vi "ctx autoconfigure devices and accesspoint5.vi"(0 "context":u32, 1 "accel_full_scale_mode":bool, 2 "enable_gyro":bool, 3 "decimation_rate":u32(ring) items=["APDM_DECIMATE_1x1", "APDM_DECIMATE_2x1", "APDM_DECIMATE_2x2", "APDM_DECIMATE_5x1", "APDM_DECIMATE_4x2", "APDM_DECIMATE_5x2", "APDM_DECIMATE_4x4", "APDM_DECIMATE_5x4", "APDM_DECIMATE_8x4", "APDM_DECIMATE_8x5", "APDM_DECIMATE_8x8"], 5 "wireless_channel_number":u8, 7 "enable_sd_card":bool, 9 "erase_sd_card":bool, 12 "enable_accel":bool, 13 "enable_mag":bool) -> (4 "context out":u32, 6 "function return":i32)   [LabVIEW 2019, in "apdm.lvlib"]
doc: "APDM_EXPORT int apdm_ctx_autoconfigure_devices_and_accesspoint5(apdm_ctx_t context, const uint8_t wireless_channel_number, const bool enable_sd_card,\n const bool erase_sd_card, const bool accel_full_scale_mode, const bool enable_accel, const bool enable_gyro, const bool enable_mag, const apdm_monitor_decimation_rate_t decimation_rate);"
uses:
  apdm.lvlib
  Lee Lab/CP FES Walking 2018/Code/Working/LabVIEW/apdm.dll
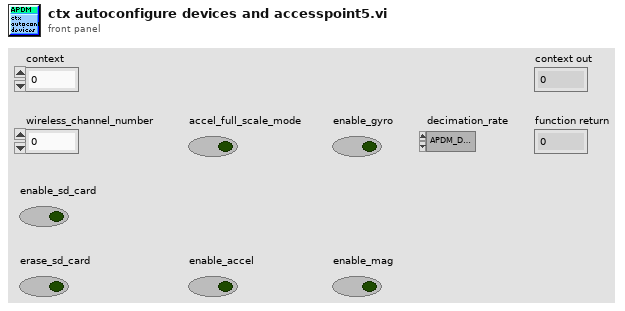
[diagram p1: front panel]
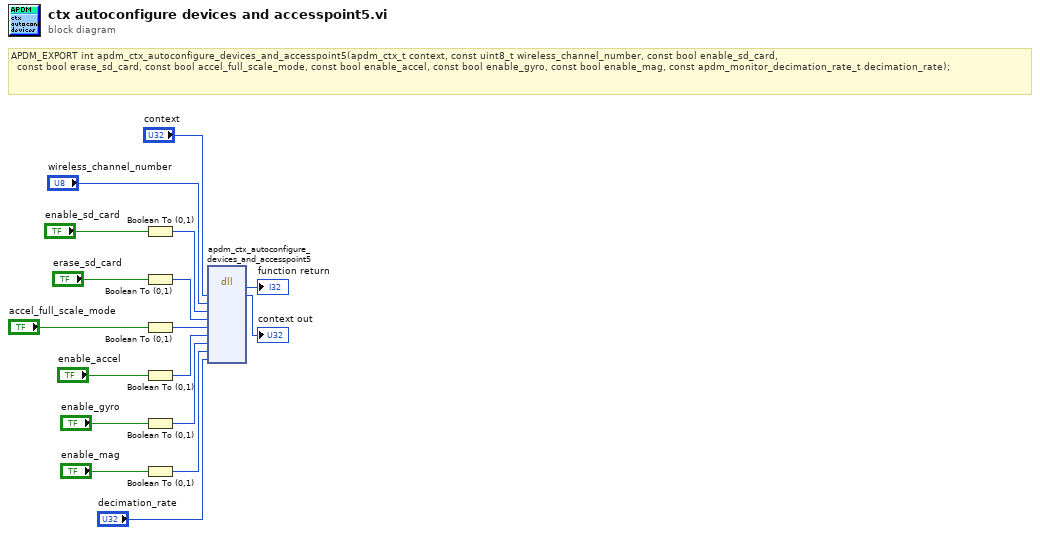
[diagram p0: block diagram]
diagram:
  # "APDM_EXPORT int apdm_ctx_autoconfigure_devices_and_accesspoint5(apdm_ctx_t context, const uint8_t wireless_channel_number, const bool enable_sd_card,\n\t\tconst bool erase_sd_card, const bool accel_full_scale_mode, const bool enable_accel, const bool enable_gyro, const bool enable_mag, const apdm_monitor_decimation_rate_t decimation_rate);"
  n1 = Boolean To (0,1)(Boolean="enable_sd_card") -> (0, 1=w12:i16)
  n2 = Boolean To (0,1)(Boolean="erase_sd_card") -> (0, 1=w10:i16)
  n3 = Boolean To (0,1)(Boolean="accel_full_scale_mode") -> (0, 1=w8:i16)
  n4 = Boolean To (0,1)(Boolean="enable_accel") -> (0, 1=w6:i16)
  n5 = Boolean To (0,1)(Boolean="enable_gyro") -> (0, 1=w4:i16)
  n6 = Boolean To (0,1)(Boolean="enable_mag") -> (0, 1=w2:i16)
  n7 = dll-call lib="C:/Users/jfalesi/Dropbox/Lee Lab/CP FES Walking 2018/Code/Working/LabVIEW/apdm.*" fn="apdm_ctx_autoconfigure_devices_and_accesspoint5"("context"="context", "wireless_channel_number"="wireless_channel_number", "enable_sd_card"=w12, "erase_sd_card"=w10, "accel_full_scale_mode"=w8, "enable_accel"=w6, "enable_gyro"=w4, "enable_mag"=w2, "decimation_rate"="decimation_rate") -> (→"function return":i32, "context"=→"context out":u32)  [unwired: 11 in, 2 out]
